vi "局部变量（一个开关控制两个循环）.vi"() -> ()   [LabVIEW 2017]
panel:
  out "数字(0-1) 2":dbl
  in  "停止":bool
  out "数字(0-1)":dbl
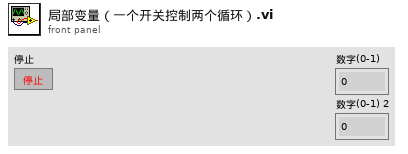
[diagram p1: front panel]
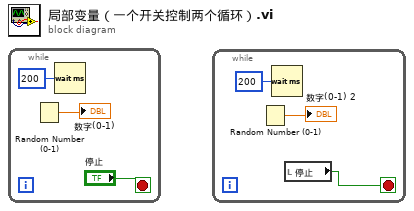
[diagram p0: block diagram]
diagram:
  n1 = while {
    stop <- "停止" stop-if-true
    n2 = Random Number (0-1)() -> (number: 0 to 1=→"数字(0-1)":dbl)
    n3 = Wait (ms)(milliseconds to wait=u32 200 ("等待时间（毫秒）")) -> ()  [unwired: 1 out]
  }
  n4 = while {
    stop <- w5 stop-if-true
    n5 = Random Number (0-1)() -> (number: 0 to 1=→"数字(0-1) 2":dbl)
    n6 = Wait (ms)(milliseconds to wait=u32 200 ("等待时间（毫秒）")) -> ()  [unwired: 1 out]
    n7 = local read "停止"() -> (w5:bool)
  }
